vi "RemoveLineBreaks.vi"(8 "error in (no error)":errorcluster, 11 "Input string":string) -> (0 "error out":errorcluster, 3 "String linefeeds removed":string)   [LabVIEW 2023, in "SimpleErrorLogger.lvlib"]
uses:
  SimpleErrorLogger.lvlib
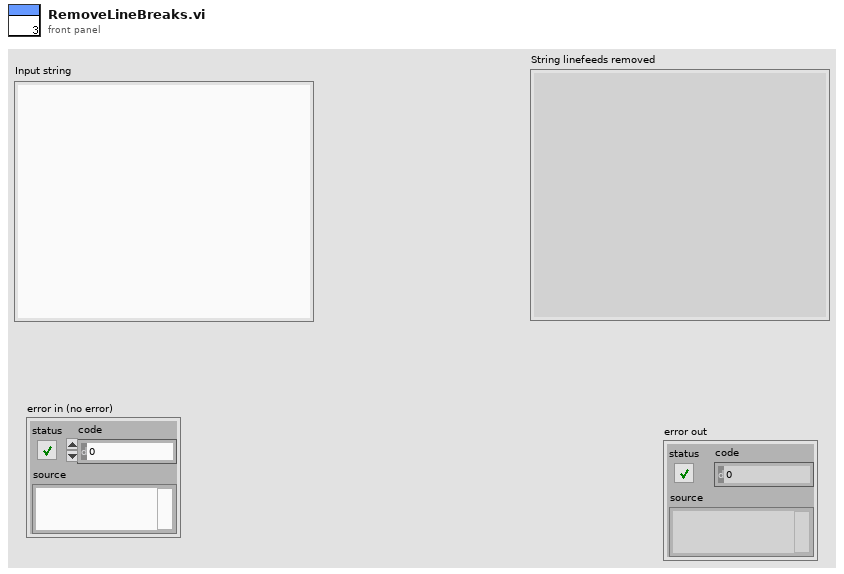
[diagram p1: front panel]
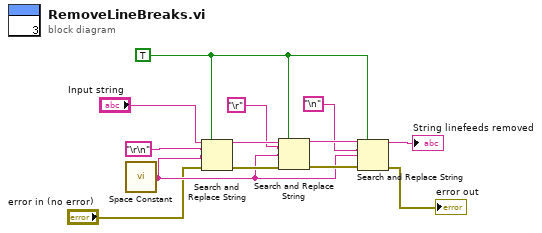
[diagram p0: block diagram]
diagram:
  w1 = TRUE ("replace all? (F)")
  n1 = call <vilib>:"Space Constant.vi"() -> ("String"=w5:string)
  n2 = Search and Replace String(replace all?=w1, input string="Input string", search string="\r\n", replace string=w5, error in="error in (no error)") -> (result string=w11:string, error out=w10:errorcluster)  [unwired: 3 in, 2 out]
  n3 = Search and Replace String(replace all?=w1, input string=w11, search string="\r", replace string=w5, error in=w10) -> (result string=w7:string, error out=w8:errorcluster)  [unwired: 3 in, 2 out]
  n4 = Search and Replace String(replace all?=w1, input string=w7, search string="\n", replace string=w5, error in=w8) -> (result string=→"String linefeeds removed":string, error out=→"error out":errorcluster)  [unwired: 3 in, 2 out]
